vi "Write Data.vi"(8 "error in (no error)":errorcluster, 9 "Data":variant, 10 "Address":string, 11 "SIMATIC_S7 in":refnum<class "SIMATIC_S7.lvclass">) -> (0 "error out":errorcluster, 3 "SIMATIC_S7 out":refnum<class "SIMATIC_S7.lvclass">)   [LabVIEW 2025, in "SIMATIC_S7.lvclass"]
uses:
  SIMATIC_S7.lvclass
  SIMATIC_S7.lvclass/SIMATIC_S7.ctl
  <vilib>/Hampel Software Engineering/S7NetCom/Source/API/Write Data - Boolean (Scalar).vi
  <vilib>/Hampel Software Engineering/S7NetCom/Source/API/Write Data - Byte (Scalar).vi
  <vilib>/Hampel Software Engineering/S7NetCom/Source/API/Write Data - Real (Scalar).vi
  <vilib>/Hampel Software Engineering/S7NetCom/Source/API/Write Data - DWord (Scalar).vi
  <vilib>/Hampel Software Engineering/S7NetCom/Source/API/Write Data - DWord (Array).vi
  <vilib>/Utility/Data Type/NI_Data Type.lvlib
  <vilib>/Hampel Software Engineering/S7NetCom/Source/S7NetCom.lvclass
  <vilib>/Hampel Software Engineering/S7NetCom/Source/API/Write Data - String.vi
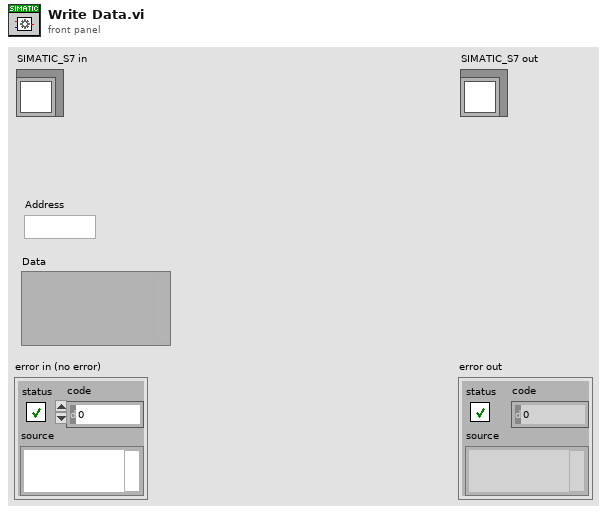
[diagram p1: front panel]
types:
  T1 = typedef "S7NetCom.lvlib/S7NetCom.lvclass/S7_Memory_Area.ctl" = enum8{"P Area", "I Area", "O Area", "M Area", "DB Area", "Counter", "Timer"}
  T2 = typedef "NI_Data Type.lvlib/Data Type.ctl" = enum8{"Invalid Type", "Void", "I8", "I16", "I32", "I64", "U8", "U16", "U32", "U64", "Single Float", "Double Float", "Extended Float", "Single Complex", "Double Complex", "Extended Complex", "Enum U8", "Enum U16", "Enum U32", "Enum U64", "Single Float With Unit", "Double Float With Unit", "Extended Float With Unit", "Single Complex with Unit", "Double Complex with Unit", "Extended Complex with Unit", "Boolean", "String", "Path", "Picture", "Tag", "Array", "Cluster", "Variant", "LV Variant", "Waveform", "Timestamp", "Digital Waveform", "Digital Data", "ExpressData", "Refnum", "External Data", "VI", "Poly VI", "LabVIEW Class Instance", "Fixed Point", "Set Collection", "Map Collection"}
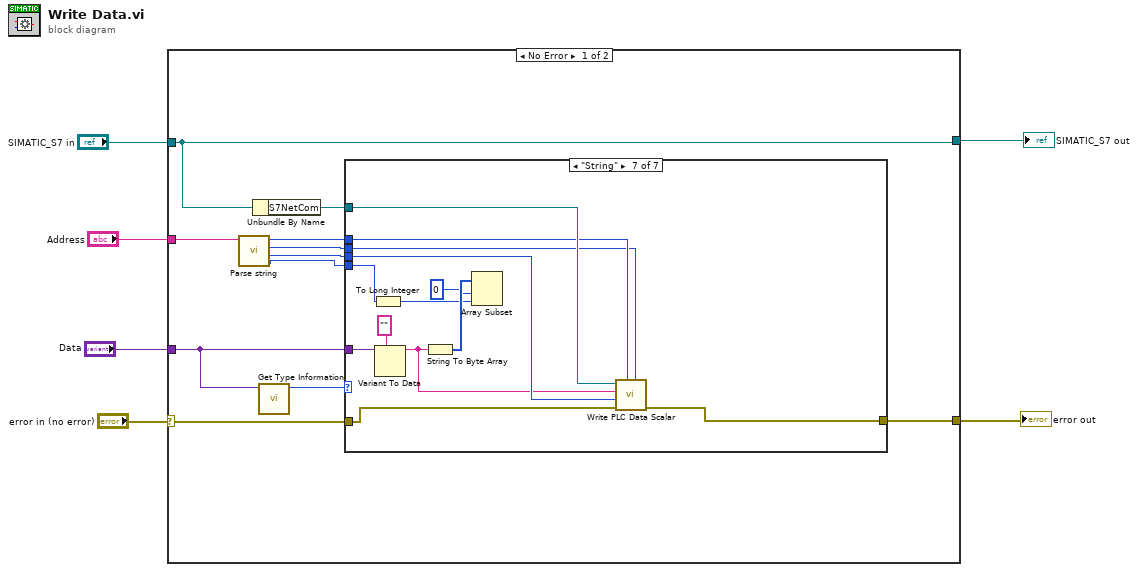
[diagram p0: block diagram]
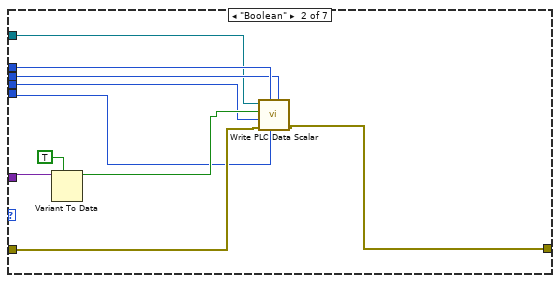
[diagram p3: hidden frame]
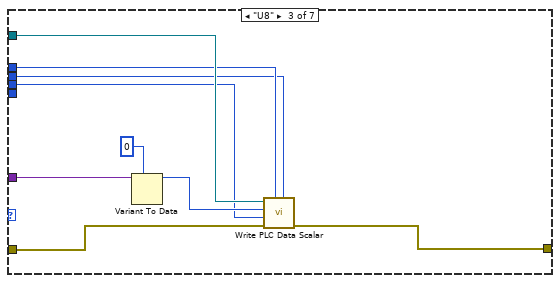
[diagram p4: hidden frame]
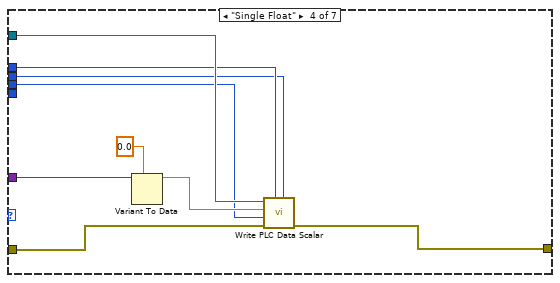
[diagram p5: hidden frame]
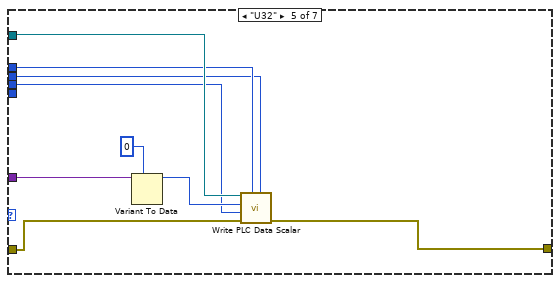
[diagram p6: hidden frame]
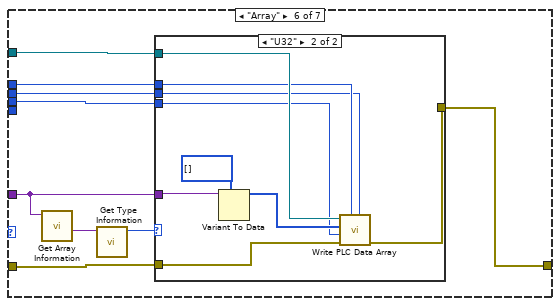
[diagram p7: hidden frame]
diagram:
  n1 = case shown="No Error" "error in (no error)" {
    selector: "error in (no error)" -> [w13 w89]
    tunnel: [w12 w89] -> w5
    tunnel: "SIMATIC_S7 in" -> [w17 w88]
    tunnel: [w17 w88] -> w3
    tunnel: "Address" -> [w11 _]
    tunnel: "Data" -> [w14 _]
    frame No Error {
      n2 = call "Parse string.vi"("Address"=w11) -> ("Len"=w7:u8, "StartAddress"=w8:u32, "DataBlock"=w9:u16, "Memory Area"=w10:T1)  [unwired: 7 in]
      n3 = Unbundle By Name(w17) -> ("S7NetCom"=w15:refnum<class "S7NetCom.lvclass">)
      n4 = call <vilib>:"Get Type Information.vi"("variant"=w14) -> ("type"=w16:T2)  [unwired: 6 in, 4 out]
      n5 = case shown="\"String\"" w16 {
        tunnel: w15 -> [_ w26 w37 w46 w55 w64 w85]
        tunnel: w14 -> [_ w25 w36 w45 w54 w59 w87]
        tunnel: w13 -> [w18 w22 w33 w42 w51 w63 w84]
        tunnel: [w18 w21 w32 w41 w50 w62 w83] -> w12
        tunnel: w10 -> [_ w28 w31 w40 w49 w58 w82]
        tunnel: w9 -> [_ w27 w30 w39 w48 w57 w81]
        tunnel: w8 -> [_ w20 w29 w38 w47 w56 w80]
        tunnel: w7 -> [_ w19 _ _ _ _ w77]
        frame Default {
        }
        frame "Boolean" {
          n6 = Variant To Data(type=TRUE, Variant=w25) -> (data=w23:bool)  [unwired: 1 in, 1 out]
          n7 = call-poly <vilib>:"Write PLC Data Scalar.vi"("Data Block #"=w27, "Bit Offset"=w19, "Memory Area"=w28, "error in (no error)"=w22, "Start Address"=w20, "Value"=w23, "S7 in"=w26) -> ("error out"=w21:errorcluster)  [unwired: 3 in, 1 out]
        }
        frame "U8" {
          n8 = Variant To Data(type=u8 0, Variant=w36) -> (data=w34:u8)  [unwired: 1 in, 1 out]
          n9 = call-poly <vilib>:"Write PLC Data Scalar.vi"("Data Block #"=w30, "Memory Area"=w31, "error in (no error)"=w33, "Start Address"=w29, "Value"=w34, "S7 in"=w37) -> ("error out"=w32:errorcluster)  [unwired: 4 in, 1 out]
        }
        frame "Single Float" {
          n10 = Variant To Data(type=sgl 0.0, Variant=w45) -> (data=w43:sgl)  [unwired: 1 in, 1 out]
          n11 = call-poly <vilib>:"Write PLC Data Scalar.vi"("Data Block #"=w39, "Memory Area"=w40, "error in (no error)"=w42, "Start Address"=w38, "Value"=w43, "S7 in"=w46) -> ("error out"=w41:errorcluster)  [unwired: 4 in, 1 out]
        }
        frame "U32" {
          n12 = Variant To Data(type=u32 0, Variant=w54) -> (data=w52:u32)  [unwired: 1 in, 1 out]
          n13 = call-poly <vilib>:"Write PLC Data Scalar.vi"("Data Block #"=w48, "Memory Area"=w49, "error in (no error)"=w51, "Start Address"=w47, "Value"=w52, "S7 in"=w55) -> ("error out"=w50:errorcluster)  [unwired: 4 in, 1 out]
        }
        frame "Array" {
          n14 = call <vilib>:"Get Array Information.vi"("variant"=w59) -> ("array element data type"=w61:variant)  [unwired: 7 in, 3 out]
          n15 = call <vilib>:"Get Type Information.vi"("variant"=w61) -> ("type"=w60:T2)  [unwired: 6 in, 4 out]
          n16 = case shown="\"U32\"" w60 {
            tunnel: w64 -> [_ w74]
            tunnel: w63 -> [w65 w72]
            tunnel: [w65 w73] -> w62
            tunnel: w59 -> [_ w71]
            tunnel: w58 -> [_ w68]
            tunnel: w57 -> [_ w67]
            tunnel: w56 -> [_ w66]
            frame Default {
            }
            frame "U32" {
              n17 = Variant To Data(type=u32[] [], Variant=w71) -> (data=w69:u32[])  [unwired: 1 in, 1 out]
              n18 = call-poly <vilib>:"Write PLC Data Array.vi"("Data Block #"=w67, "Memory Area"=w68, "error in (no error)"=w72, "Start Address"=w66, "DWord Array"=w69, "S7 in"=w74) -> ("error out"=w73:errorcluster)  [unwired: 4 in, 1 out]
            }
          }
        }
        frame "String" {
          n19 = To Long Integer(number=w77) -> (32bit integer=w76:i32)
          n20 = Variant To Data(type="", Variant=w87) -> (data=w75:string)  [unwired: 1 in, 1 out]
          n21 = String To Byte Array(string=w75) -> (unsigned byte array=w79:u8[])
          n22 = Array Subset(array=w79, index=0, length=w76) -> ()  [unwired: 1 out]
          n23 = call-poly <vilib>:"Write PLC Data Scalar.vi"("Data Block #"=w81, "Memory Area"=w82, "error in (no error)"=w84, "Start Address"=w80, "String"=w75, "S7 in"=w85) -> ("error out"=w83:errorcluster)  [unwired: 4 in, 1 out]
        }
      }
    }
    frame Error {
    }
  }
  "error out" <- w5
  "SIMATIC_S7 out" <- w3
